vi "Init Device.vi"(7 "Layout Ref":refnum<vi>, 8 "error in (no error)":errorcluster, 10 "Chan# Array":i32[](array[numeric]), 11 "DDS in":refnum<class "DDS.lvclass">) -> (0 "error out":errorcluster, 3 "DDS out":refnum<class "DDS.lvclass">)   [LabVIEW 2013, in "DDS.lvclass"]
doc: "Initialize the correct columns and their default appearance. If the Chan# Array is [3] or [5], the correct columns are initialized for non-sweeps or sweeps mode WITHOUT touching the Device Settings bools. Otherwise, Sweeps ON is assumed and ALL front panel default values are used.\n\nUse this front panel to change default appearance of the device in the Add/Manage devices or Load from Old."
uses:
  DDS.lvclass
  ColumnVIs/Column/Column.lvclass
  ColumnVIs/DigitalCol/DigitalCol.lvclass
  TypeDefs/ColumnAppearCluster.ctl
  TypeDefs/DigitalColumnAppearCluster.ctl
  DDS.lvclass/DDS.ctl
panel:
  in  "Setup":T1={"PB trig / Sequence"=TRUE, "Amp Lock?"=FALSE}
  in  "Sweep Dir. Column Defaults":T2={"Column Name"="", "Width"=18, "Bkgd"=[1985280, 6618880, 14090026], "Text"=[16448250, 0, 0]}
  in  "Amp Column Defaults":T3={"Column Name"="", "Width"=30, "Bkgd"=[16448250], "Text"=[0]}
  in  "Phase Column Defaults":T3={"Column Name"="", "Width"=30, "Bkgd"=[16448250], "Text"=[0]}
  in  "Freq 0/1 Column Defaults":T3={"Column Name"="", "Width"=30, "Bkgd"=[16448250], "Text"=[0]}
  # "Need Sweeps ON by default so that we\ncan create all 5 possible column types."
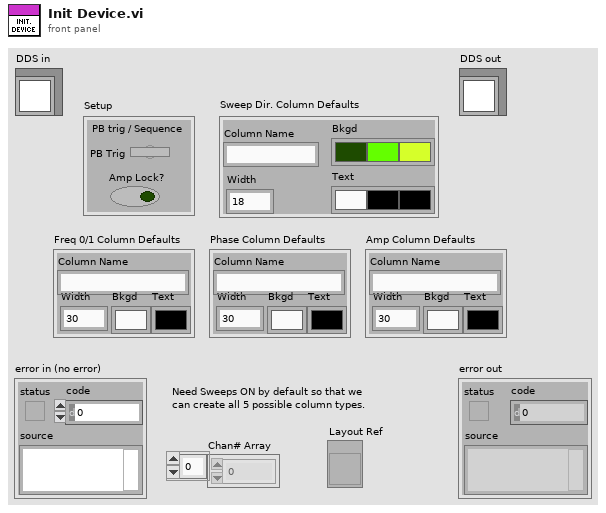
[diagram p1: front panel]
types:
  T1 = cluster{"PB trig / Sequence":bool, "Amp Lock?":bool}
  T2 = typedef "DigitalColumnAppearCluster.ctl" = cluster{"Column Name":string, "Width":u32, "Bkgd":u32[], "Text":u32[]}
  T3 = typedef "ColumnAppearCluster.ctl" = cluster{"Column Name":string, "Width":u32, "Bkgd":u32[], "Text":u32[]}
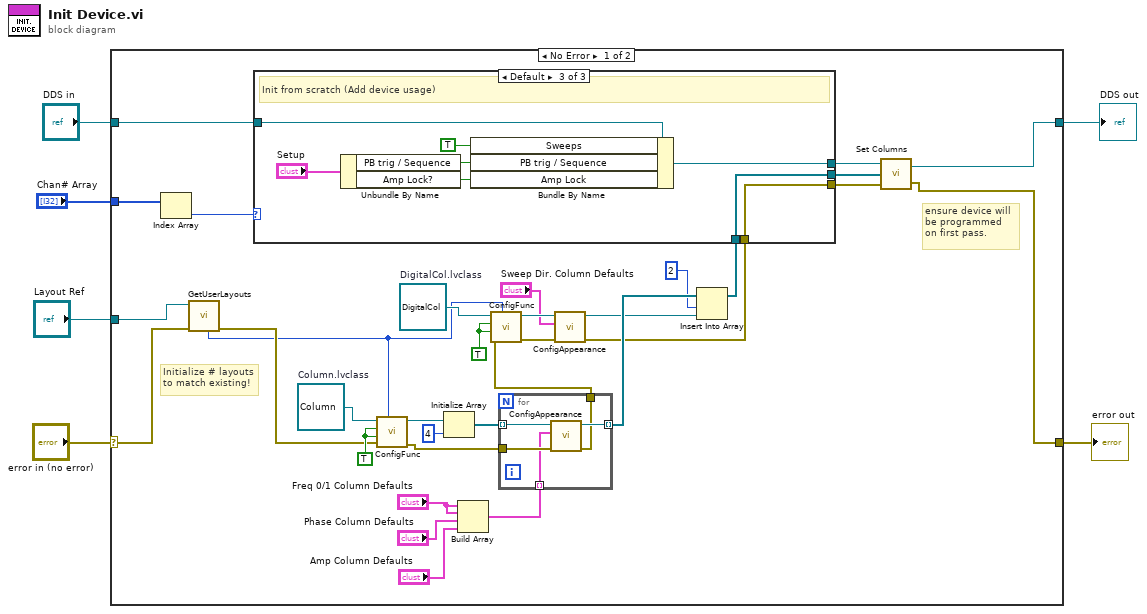
[diagram p0: block diagram]
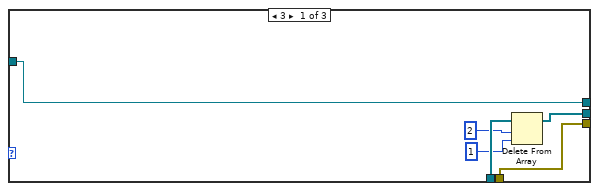
[diagram p2: hidden frame]
diagram:
  n1 = case shown="No Error" "error in (no error)" {
    selector: "error in (no error)" -> [w12 w62]
    tunnel: "DDS in" -> [w39 w63]
    tunnel: [w8 w63] -> w3
    tunnel: [w7 w62] -> w4
    tunnel: "Layout Ref" -> [w9 _]
    tunnel: "Chan# Array" -> [w18 _]
    frame No Error {
      w36 = TRUE ("Disableable? (True)")
      w37 = TRUE ("Disableable? (True)")
      w35 = refnum<class "DigitalCol.lvclass"> refnum  # DigitalCol.lvclass
      w38 = refnum<class "Column.lvclass"> refnum  # Column.lvclass
      # "ensure device will\nbe programmed\non first pass."
      # "Initialize # layouts\nto match existing!"
      n2 = Index Array(array=w18) -> (element=w13:i32)  [unwired: 1 in]
      n3 = call "GetUserLayouts.vi"("error in (no error)"=w12, "Layout Ring Refnum"=w9) -> ("error out"=w11:errorcluster, "Num User Layouts"=w10:i32)  [unwired: 5 in, 3 out]
      n4 = call "ConfigFunc.vi"("Num Layouts (ignored)"=w10, "error in (no error)"=w11, "isVariable? (True)"=w37, "Disableable? (True)"=w37, "Column in"=w38) -> ("error out"=w27:errorcluster, "Column out"=w34:refnum<class "Column.lvclass">)  [unwired: 5 in]
      n5 = Initialize Array(w34, 4 ("dimension size")) -> (w28:refnum<class "Column.lvclass">[])
      n6 = Build Array("Freq 0/1 Column Defaults", "Freq 0/1 Column Defaults", "Phase Column Defaults", "Amp Column Defaults") -> (w26:T3[])
      n7 = for {
        tunnel: w28 -> [w61] mode=indexing
        tunnel: w27 -> [w60]
        tunnel: w26 -> [w59] mode=indexing
        tunnel: [w58] -> w25 mode=indexing
        tunnel: [w57] -> w19
        n8 = call "ConfigAppearance.vi"("error in (no error)"=w60, "Column Appearance"=w59, "Column in"=w61) -> ("error out"=w57:errorcluster, "Column out"=w58:refnum<class "Column.lvclass">)  [unwired: 7 in]
      }
      n9 = call "ConfigFunc.vi"("Num Layouts (ignored)"=w10, "error in (no error)"=w19, "isVariable? (True)"=w36, "Disableable? (True)"=w36, "Column in"=w35) -> ("error out"=w22:errorcluster, "Column out"=w23:refnum<class "DigitalCol.lvclass">)  [unwired: 5 in]
      n10 = call "ConfigAppearance.vi"("error in (no error)"=w22, "Column Appearance"="Sweep Dir. Column Defaults", "Column in"=w23) -> ("error out"=w14:errorcluster, "Column out"=w20:refnum<class "DigitalCol.lvclass">)  [unwired: 7 in]
      n11 = Insert Into Array(array=w25, index=2, new element=w20) -> (w16:refnum<class "Column.lvclass">[])
      n12 = case shown="Default" w13 {
        tunnel: w39 -> [w45 w48 w55]
        tunnel: [w45 w48 w54] -> w32
        tunnel: [w42 w47 w50] -> w17
        tunnel: w16 -> [w43 w47 w50]
        tunnel: [w44 w46 w49] -> w15
        tunnel: w14 -> [w44 w46 w49]
        frame 3 {
          n13 = Delete From Array(array=w43, length=2, index=1) -> (array with subset deleted=w42:refnum<class "Column.lvclass">[])  [unwired: 1 out]
        }
        frame 5 {
        }
        frame Default {
          # "Init from scratch (Add device usage)"
          n14 = Unbundle By Name("Setup") -> ("PB trig / Sequence"=w52:bool, "Amp Lock?"=w51:bool)
          n15 = Bundle By Name(cluster=w55, "Sweeps"=TRUE ("AO Channel.Sweeps"), "PB trig / Sequence"=w52, "Amp Lock"=w51) -> (w54:refnum<class "DDS.lvclass">)
        }
      }
      n16 = call-dynamic "Set Columns.vi"("error in (no error)"=w15, "Columns in"=w17, "DDS in"=w32) -> ("error out"=w7:errorcluster, "DDS out"=w8:refnum<class "DDS.lvclass">)  [unwired: 1 in]
    }
    frame Error {
    }
  }
  "error out" <- w4
  "DDS out" <- w3
